vi "Ack Completion Long Exec Meth.vi"(8 "error in (no error)":errorcluster, 10 "Completion Ack Data":T1, 11 "Async Methods Actor Example in":refnum<class "Async Methods Actor Example.lvclass">) -> (0 "error out":errorcluster, 3 "Async Methods Actor Example out":refnum<class "Async Methods Actor Example.lvclass">)   [LabVIEW 2023, in "Async Methods Actor Example.lvlib" / "Async Methods Actor Example.lvclass"]
uses:
  Async Methods Actor Example.lvclass
  <vilib>/LS Instruments AG/Async Methods Actor/Async Methods Actor/Async Methods Actor Messages/Completion Notification Msg/Completion Notification Data.ctl
  <vilib>/LS Instruments AG/Async Methods Actor/Async Methods Actor/Async Methods Actor Messages/Async Message/Async Message.lvclass
  Async Methods Actor Example.lvclass/Async Methods Actor Example.ctl
  <vilib>/LS Instruments AG/Async Methods Actor/Async Methods Actor/Async Methods Actor Messages/Completion Notification Msg/Completion Notification Msg.lvclass
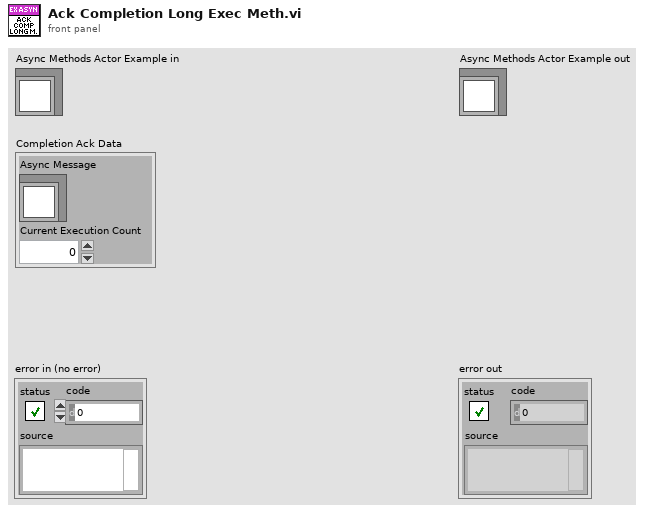
[diagram p1: front panel]
types:
  T1 = typedef "Async Methods Actor.lvlib/Completion Notification Msg.lvclass/Completion Notification Data.ctl" = cluster{"Async Message":refnum<class "Async Message.lvclass">, "Current Execution Count":u32}
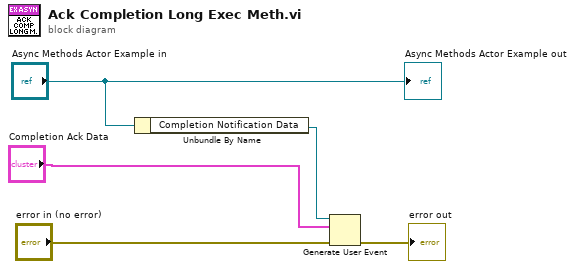
[diagram p0: block diagram]
diagram:
  n1 = Unbundle By Name("Async Methods Actor Example in") -> ("Completion Notification Data"=w3:refnum<user-event>)
  n2 = Generate User Event(user event=w3, event data cluster="Completion Ack Data", error in="error in (no error)") -> (error out=→"error out":errorcluster)  [unwired: 1 in, 1 out]
  "Async Methods Actor Example out" <- "Async Methods Actor Example in"
